vi "Example7-Interfaces.vi"   [LabVIEW 2021]
doc: "Example of useing interfaces in LabVIEW. Comments in Polish."
uses:
  Jedi/Jedi.lvclass
  Spaceship/Spaceship.lvclass
  Debug/Debug.lvclass
  Astromech droid/Astromech droid.lvclass
  Droid/Droid.lvclass
  LogClassData/LogClassData.lvclass
  MulitInterface/MulitInterface.lvclass
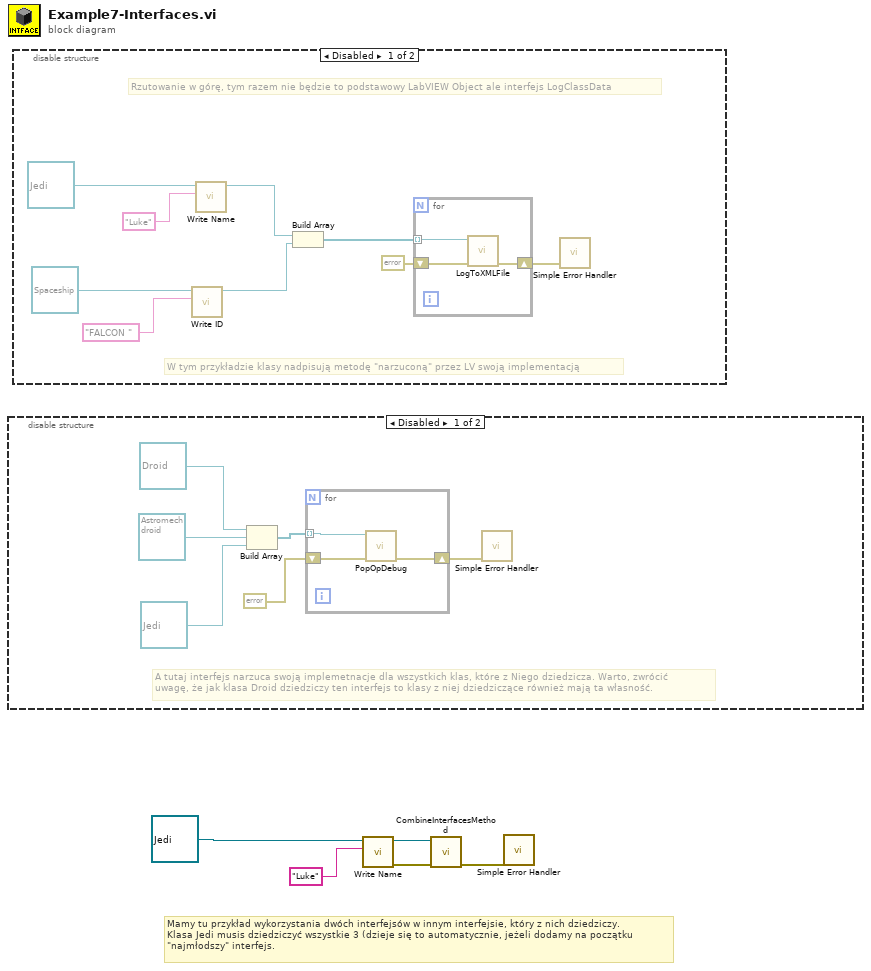
[diagram p0: block diagram]
diagram:
  # "Mamy tu przykład wykorzystania dwóch interfejsów w innym interfejsie, który z nich dziedziczy. \nKlasa Jedi musis dziedziczyć wszystkie 3 (dzieje się to automatycznie, jeżeli dodamy na początku \n\"najmłodszy\" interfejs."
  n1 = disable-structure shown="Disabled" {
    frame Disabled {
      # "A tutaj interfejs narzuca swoją implemetnacje dla wszystkich klas, które z Niego dziedzicza. Warto, zwrócić \nuwagę, że jak klasa Droid dziedziczy ten interfejs to klasy z niej dziedziczące również mają ta własność."
      n2 = Build Array(refnum<class "Droid.lvclass"> refnum ("Droid.lvclass"), refnum<class "Astromech droid.lvclass"> refnum ("Astromech droid.lvclass"), refnum<class "Jedi.lvclass"> refnum ("Jedi.lvclass")) -> (w10:refnum<class "Debug.lvclass">[])
      n3 = for {
        tunnel: w10 -> [w14] mode=indexing
        shift-right: [w13] -> w7
        shift-left: errorcluster {"status"=FALSE, "code"=0, "source"=""} ("Error Out") -> [w12]
        n4 = call "PopOpDebug.vi"("Error In"=w12, "Debug in"=w14) -> ("Error Out"=w13:errorcluster)  [unwired: 8 in, 1 out]
      }
      n5 = call <vilib>:"Simple Error Handler.vi"("error in (no error)"=w7) -> ()  [unwired: 4 in, 5 out]
    }
    frame Enabled {
    }
  }
  n6 = disable-structure shown="Disabled" {
    frame Disabled {
      # "W tym przykładzie klasy nadpisują metodę \"narzuconą\" przez LV swoją implementacją"
      # "Rzutowanie w górę, tym razem nie będzie to podstawowy LabVIEW Object ale interfejs LogClassData"
      n7 = call-dynamic "Write ID.vi"("ID"="FALCON ", "Spaceship in"=refnum<class "Spaceship.lvclass"> refnum ("Spaceship.lvclass")) -> ("Spaceship out"=w18:refnum<class "Spaceship.lvclass">)  [unwired: 8 in, 1 out]
      n8 = call-dynamic "Write Name.vi"("Name"="Luke", "Jedi in"=refnum<class "Jedi.lvclass"> refnum ("Jedi.lvclass")) -> ("Jedi out"=w19:refnum<class "Jedi.lvclass">)  [unwired: 8 in, 1 out]
      n9 = Build Array(w19, w18) -> (w17:refnum<class "LogClassData.lvclass">[])
      n10 = for {
        tunnel: w17 -> [w26] mode=indexing
        shift-right: [w25] -> w15
        shift-left: errorcluster {"status"=FALSE, "code"=0, "source"=""} ("Error Out") -> [w24]
        n11 = call-dynamic "LogToXMLFile.vi"("Error In"=w24, "LogClassData In"=w26) -> ("Error Out"=w25:errorcluster)  [unwired: 8 in, 1 out]
      }
      n12 = call <vilib>:"Simple Error Handler.vi"("error in (no error)"=w15) -> ()  [unwired: 4 in, 5 out]
    }
    frame Enabled {
    }
  }
  n13 = call-dynamic "Write Name.vi"("Name"="Luke", "Jedi in"=refnum<class "Jedi.lvclass"> refnum ("Jedi.lvclass")) -> ("error out"=w2:errorcluster, "Jedi out"=w1:refnum<class "Jedi.lvclass">)  [unwired: 8 in]
  n14 = call "CombineInterfacesMethod.vi"("Error In"=w2, "MulitInterface In"=w1) -> ("Error Out"=w5:errorcluster)  [unwired: 8 in, 1 out]
  n15 = call <vilib>:"Simple Error Handler.vi"("error in (no error)"=w5) -> ()  [unwired: 4 in, 5 out]
